vi "sub_VI.vi"(11 "Ctl 참조 번호":refnum<vi>) -> ()   [LabVIEW 2020]
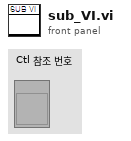
[diagram p1: front panel]
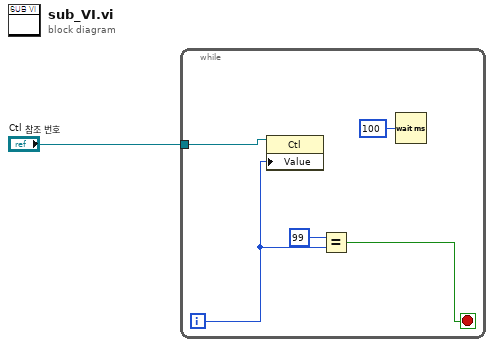
[diagram p0: block diagram]
diagram:
  n1 = while {
    tunnel: "Ctl 참조 번호" -> [w6]
    i -> [w5]
    stop <- w3 stop-if-true
    n2 = property class="Ctl"(reference=w6, "Value"=w5) -> ()  [unwired: 1 in, 2 out]
    n3 = Equal?(x=99, y=w5) -> (x = y?=w3:bool)
    n4 = Wait (ms)(milliseconds to wait=u32 100 ("대기 시간 (ms)")) -> ()  [unwired: 1 out]
  }
